vi "Wait.vi"() -> ()   [LabVIEW 2017]
panel:
  in  "Time":u32
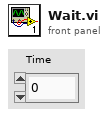
[diagram p1: front panel]
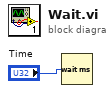
[diagram p0: block diagram]
diagram:
  n1 = Wait (ms)(milliseconds to wait="Time") -> ()  [unwired: 1 out]
